vi "wrapper Init.vi"(0 "dim":i32, 1 "fileName":string, 2 "discType":string, 3 "upwindType":string, 4 "subsets":string, 5 "setDiffusionValue":bool, 6 "diffusionValue":dbl, 7 "error in (no error)":errorcluster, 8 "diffusionMatrix":dbl[][](array[numeric])=[[0.0, 0.0, 0.0]], 9 "reactionRateValue":dbl, 10 "sourceValue":dbl, 11 "massScaleValue":dbl, 12 "velocityVector":dbl[](array[numeric])=[0.0, 0.0, 0.0], 13 "precondName":string, 14 "solverName":string, 15 "numRefs":i32, 16 "maxNumIter":i32, 17 "absTol":dbl) -> (20 "velocityVector out":dbl[](array[numeric]), 21 "function return":i32, 27 "error out":errorcluster)   [LabVIEW 2019, in "libConvectionDiffusionWrapper.lvlib"]
doc: "int wrapperInit(\n int dim, \n const char* fileName,\n const char* discType, \n const char* upwindType, \n const char* subsets,\n bool setDiffusionValue,\n double diffusionValue,\n double diffusionMatrix[3][3], \n double reactionRateValue,\n double sourceValue,\n double massScaleValue,\n double velocityVector[3][1],\n const char* precondName,\n const char* solverName,\n int numRefs,\n int maxNumIter,\n double absTol)"
uses:
  libConvectionDiffusionWrapper.lvlib
panel:
  out "diffusionMatrix out":dbl[][](array[numeric])
  # "******************************************************************\n*** Convection Diffusion Application\n******************************************************************\nAuthor: Paul Zügel\nGCSC - Frankfurt 2020"
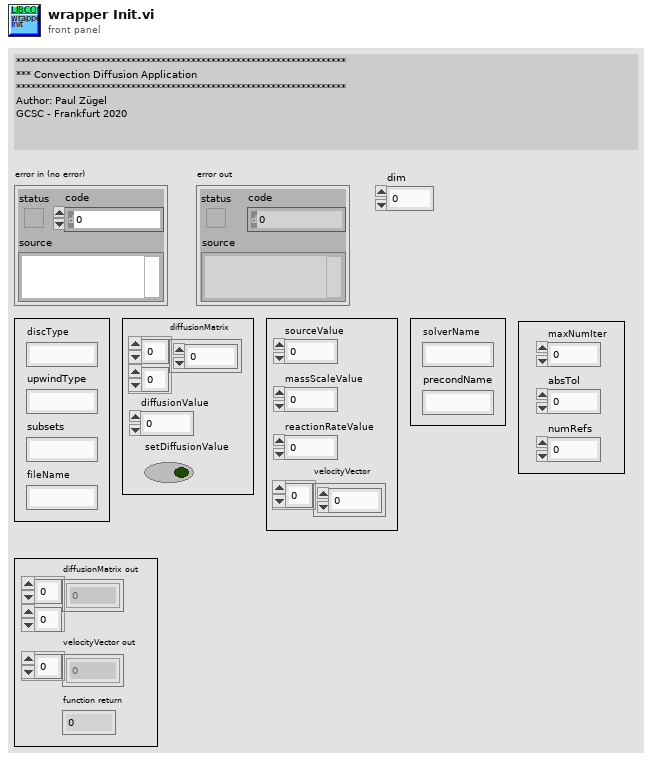
[diagram p1: front panel]
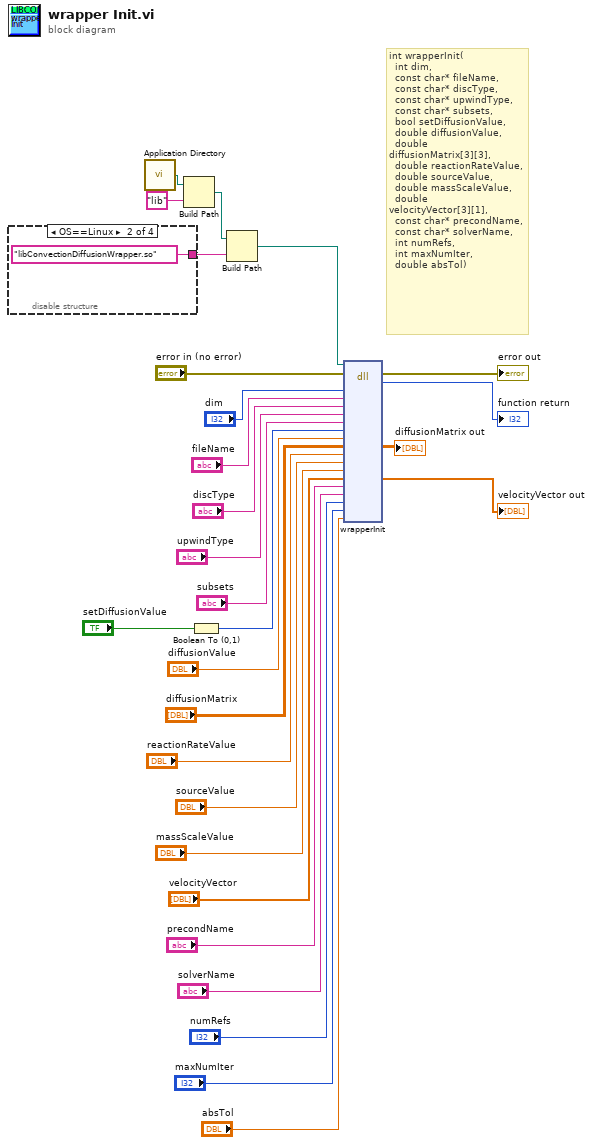
[diagram p0: block diagram]
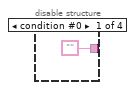
[diagram p2: hidden frame]
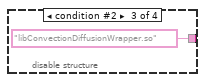
[diagram p3: hidden frame]
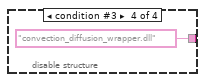
[diagram p4: hidden frame]
diagram:
  # "int wrapperInit(\n\t\tint dim, \n\t\tconst char* fileName,\n\t\tconst char* discType, \n\t\tconst char* upwindType, \n\t\tconst char* subsets,\n\t\tbool setDiffusionValue,\n\t\tdouble diffusionValue,\n\t\tdouble diffusionMatrix[3][3],\t\n\t\tdouble reactionRateValue,\n\t\tdouble sourceValue,\n\t\tdouble massScaleValue,\n\t\tdouble velocityVector[3][1],\n\t\tconst char* precondName,\n\t\tconst char* solverName,\n\t\tint numRefs,\n\t\tint maxNumIter,\n\t\tdouble absTol)"
  n1 = disable-structure shown="OS==Linux" {
    disable-tunnel: ["" "libConvectionDiffusionWrapper.so" ("name or relative path") "libConvectionDiffusionWrapper.so" ("name or relative path") "convection_diffusion_wrapper.dll" ("name or relative path")] -> w2
    frame condition #0 {
    }
    frame condition #1 (active) {
    }
    frame condition #2 {
    }
    frame condition #3 {
    }
  }
  n2 = call <vilib>:"Application Directory.vi"() -> ("Application Directory"=w5:path)
  n3 = Build Path(base path=w5, name or relative path="lib") -> (appended path=w3:path)
  n4 = Boolean To (0,1)(Boolean="setDiffusionValue") -> (0, 1=w21:i16)
  n5 = Build Path(base path=w3, name or relative path=w2) -> (appended path=w1:path)
  n6 = dll-call lib="home/paul/Schreibtisch/Convection_diffusion/LabView/lib/libConvectionDiffusionWrapper.*" fn="wrapperInit"(path in=w1, error in="error in (no error)", "dim"="dim", "fileName"="fileName", "discType"="discType", "upwindType"="upwindType", "subsets"="subsets", "setDiffusionValue"=w21, "diffusionValue"="diffusionValue", "diffusionMatrix"="diffusionMatrix", "reactionRateValue"="reactionRateValue", "sourceValue"="sourceValue", "massScaleValue"="massScaleValue", "velocityVector"="velocityVector", "precondName"="precondName", "solverName"="solverName", "numRefs"="numRefs", "maxNumIter"="maxNumIter", "absTol"="absTol") -> (error out=→"error out":errorcluster, "return type"=→"function return":i32, "diffusionMatrix"=→"diffusionMatrix out":dbl[][], "velocityVector"=→"velocityVector out":dbl[])  [unwired: 16 in, 1 out]
